vi "_REP_BackLabel.vi"(11 "label":string) -> (3 "String":string)   [LabVIEW 2017]
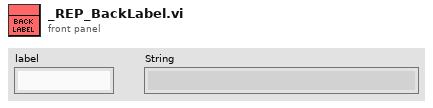
[diagram p1: front panel]
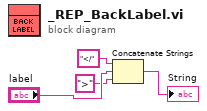
[diagram p0: block diagram]
diagram:
  n1 = Concatenate Strings("</" ("regular expression"), "label", ">" ("regular expression")) -> (→"String":string)
